vi "Control Enable.vi"(8 "error in (no error)":errorcluster, 10 "Enum":enum16{"Enb", "Dis", "Dis&G"}(ring), 11 "Reference Array":refnum<vi>[](array[refnum])) -> (0 "error out":errorcluster)   [LabVIEW 2014]
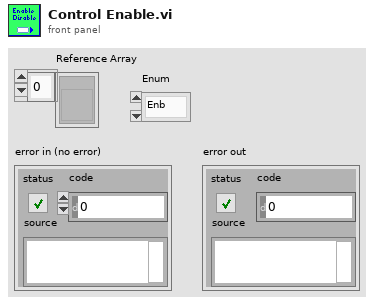
[diagram p1: front panel]
types:
  T1 = enum8{"Enabled", "Disabled", "Disabled and Grayed Out"}
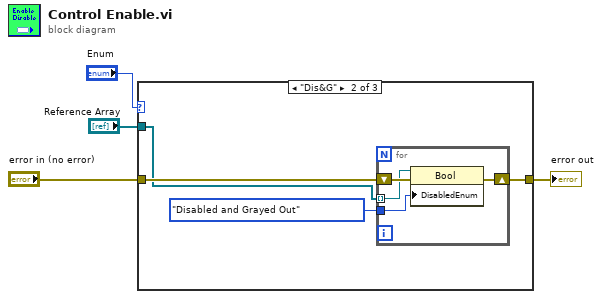
[diagram p0: block diagram]
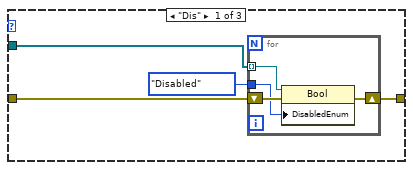
[diagram p2: hidden frame]
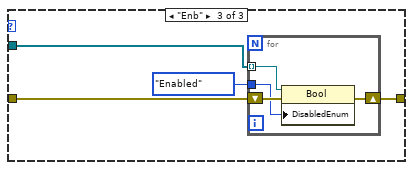
[diagram p3: hidden frame]
diagram:
  n1 = case shown="\"Dis&G\"" "Enum" {
    tunnel: [w8 w16 w24] -> w4
    tunnel: "error in (no error)" -> [w7 w15 w23]
    tunnel: "Reference Array" -> [w5 w13 w21]
    frame "Dis" {
      n2 = for {
        shift-right: [w11] -> w8
        shift-left: w7 -> [w12]
        tunnel: w5 -> [w10] mode=indexing
        tunnel: T1."Disabled" ("Disabled") -> [w9]
        n3 = property class="Bool"(reference=w10, error in=w12, "DisabledEnum"=w9) -> (error out=w11:errorcluster)  [unwired: 1 out]
      }
    }
    frame "Dis&G" {
      n4 = for {
        shift-right: [w19] -> w16
        shift-left: w15 -> [w20]
        tunnel: w13 -> [w18] mode=indexing
        tunnel: T1."Disabled and Grayed Out" ("Disabled") -> [w17]
        n5 = property class="Bool"(reference=w18, error in=w20, "DisabledEnum"=w17) -> (error out=w19:errorcluster)  [unwired: 1 out]
      }
    }
    frame "Enb" {
      n6 = for {
        shift-right: [w27] -> w24
        shift-left: w23 -> [w28]
        tunnel: w21 -> [w26] mode=indexing
        tunnel: T1."Enabled" ("Disabled") -> [w25]
        n7 = property class="Bool"(reference=w26, error in=w28, "DisabledEnum"=w25) -> (error out=w27:errorcluster)  [unwired: 1 out]
      }
    }
  }
  "error out" <- w4
